vi "CC WebRelay Test Program.vi"(8 "error in (no error)":errorcluster) -> (0 "error out":errorcluster)   [LabVIEW 2021]
uses:
  CC WebRelay enum Actions.ctl
panel:
  out "status":bool[](array[boolean])
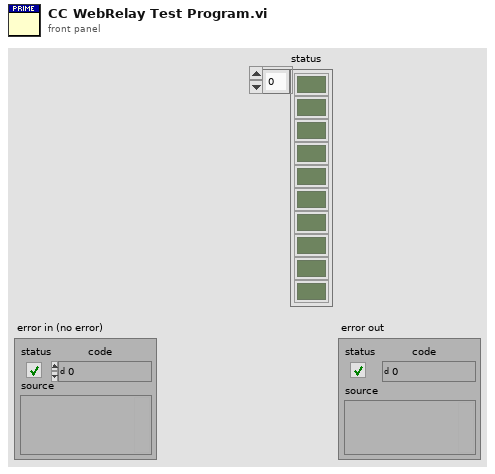
[diagram p1: front panel]
types:
  T1 = typedef "CC WebRelay enum Actions.ctl" = enum16{"Init", "Read Status", "Set Relay", "Close"}
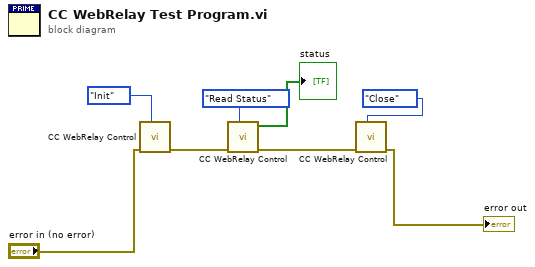
[diagram p0: block diagram]
diagram:
  n1 = call "CC WebRelay Control.vi"("Action"=CC_WebRelay_enum_Actions."Init", "error in (no error)"="error in (no error)") -> ("error out"=w6:errorcluster)  [unwired: 8 in, 1 out]
  n2 = call "CC WebRelay Control.vi"("Action"=CC_WebRelay_enum_Actions."Read Status", "error in (no error)"=w6) -> ("error out"=w5:errorcluster, "status"=→"status":bool[])  [unwired: 8 in]
  n3 = call "CC WebRelay Control.vi"("Action"=CC_WebRelay_enum_Actions."Close", "error in (no error)"=w5) -> ("error out"=→"error out":errorcluster)  [unwired: 8 in, 1 out]
